vi "Alias Already Exists.vi"() -> (2 "Error":errorcluster)   [LabVIEW 2020, in "jettl.lvlib"]
uses:
  jettl.lvlib
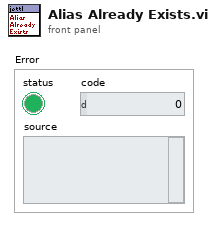
[diagram p1: front panel]
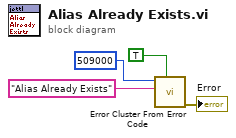
[diagram p0: block diagram]
diagram:
  n1 = call <vilib>:"Error Cluster From Error Code.vi"("show call chain? (False)"=TRUE, "error message (\"\")"="Alias Already Exists" ("Prefix"), "error code (0)"=509000) -> ("error out"=→"Error":errorcluster)  [unwired: 6 in]
